vi "TransferDataToServerComm.vi"(8 "error in (no error)":errorcluster, 10 "data":variant, 11 "Qbus":refnum<class "Qbus.lvclass">) -> (0 "error out":errorcluster)   [LabVIEW 2017, in "FileManager.lvlib"]
uses:
  <vilib>/addons/InsightCM/Devices/Shared/Common/FileManager/FileManager.lvlib
  <vilib>/addons/Qbus/Qbus.lvclass
  <vilib>/addons/InsightCM/Devices/Shared/Common/ServerComm/ServerComm.lvlib
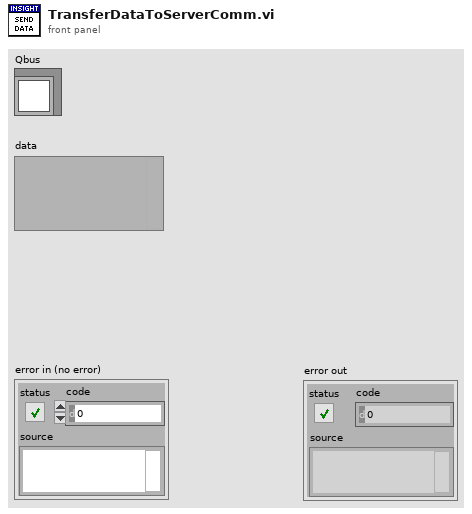
[diagram p1: front panel]
types:
  T1 = typedef "FileManager.lvlib/DataType.ctl" = enum16{"Default", "File", "InMemory", "EventRef", "EventRefFile"}
  T2 = typedef "DataEvent.lvlib/EventReference.ctl" = refnum<data-value>
  T3 = typedef "KeyValuePair.ctl" = cluster{"Key":string, "Value":string}
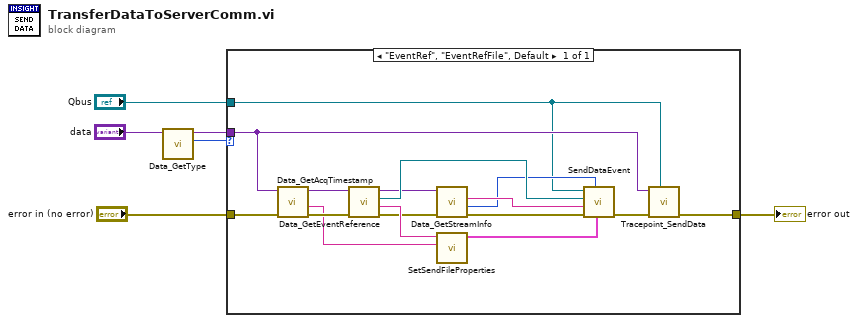
[diagram p0: block diagram]
diagram:
  n1 = call <vilib>:"Data_GetType.vi"("data"="data") -> ("type"=w4:T1, "data out"=w2:variant)  [unwired: 7 in, 2 out]
  n2 = case shown="\"EventRef\", \"EventRefFile\", Default" w4 {
    tunnel: "error in (no error)" -> [w19]
    tunnel: w2 -> [w8]
    tunnel: "Qbus" -> [w7]
    tunnel: [w10] -> w1
    frame "EventRef", "EventRefFile", Default {
      n3 = call <vilib>:"Data_GetAcqTimestamp.vi"("error in (no error)"=w19, "data"=w8) -> ("error out"=w18:errorcluster, "timestamp"=w16:string, "data out"=w17:variant)  [unwired: 6 in, 1 out]
      n4 = call <vilib>:"Data_GetEventReference.vi"("error in (no error)"=w18, "data"=w17) -> ("error out"=w15:errorcluster, "data group"=w21:string, "event reference"=w22:T2, "data out"=w13:variant)  [unwired: 4 in, 2 out]
      n5 = call <vilib>:"Data_GetStreamInfo.vi"("error in (no error)"=w15, "data"=w13) -> ("error out"=w14:errorcluster, "block"=w11:i32, "stream Id"=w12:string)  [unwired: 6 in, 1 out]
      n6 = call <vilib>:"SetSendFileProperties.vi"("acqusition timestamp"=w16, "data group"=w21) -> ("send file properties"=w20:T3[])  [unwired: 9 in]
      n7 = call <vilib>:"SendDataEvent.vi"("properties"=w20, "block"=w11, "error in (no error)"=w14, "stream id"=w12, "event reference"=w22, "Qbus in"=w7) -> ("error out"=w9:errorcluster)  [unwired: 4 in, 1 out]
      n8 = call <vilib>:"Tracepoint_SendData.vi"("Qbus in"=w7, "error in (no error)"=w9, "data in"=w8) -> ("error out"=w10:errorcluster)  [unwired: 8 in]
    }
  }
  "error out" <- w1
